vi "GageTransfer.vi"(6 "Length (4096)":dbl=4096.0, 7 "Start (0)":dbl, 8 "Segment (1)":u32=1, 9 "Mode (0)":u32 step=1, 10 "Channel (0)":u16 step=1, 11 "Handle Cluster":T1) -> (0 "Error Code":i32, 1 "Actual Length":dbl, 2 "Data_Raw":i32[](array[numeric]), 3 "Actual Start":dbl)   [LabVIEW 2013]
doc: "This VI transfers the data from one channel of the CompuScope system identified by Handle Cluster, which is obtained by calling CsTool-GetSystem.vi. For accurate interpretation of the transferred data, the user should always use the returned Actual Start and Actual Length, and not the requested values. \n\nThis VI can be used for transferring data from 8, 12, 14, and 16 bit CompuScope hardware. Data are transferred from on-board CompuScope memory to PC RAM using PCI Bus Mastering at rates of up to 200 MB/s. \n\nInternally, CsTool-Transfer.vi converts the raw integer ADC code values into double variable voltage values. For more rapid data access, the user may remove the voltage conversion step. The VI will not return programmatic control to LabVIEW until all of the data have been transferred. \n\nIf the call is successful, a 1 is returned in the Error Code indicator. If the call is unsuccessful, an appropriate error code is returned. A descriptive error string may be obtained by calling CsTool-ErrorHandler.vi.\n\n\nInput Value Descriptions:\n\nChannel\nThis integer value specifies the channel from which data are to be transferred. The default value is 0 for the first channel in the CompuScope system. Channels in a LabVIEW CompuScope system begin at 0. If an invalid channel number is given, an error will be returned. Please see the CompuScope hardware manual for more information on channel enumeration.\n\nMode\nThis integer value determines the current transfer mode. Currently, the only valid value for this input is 0.\n\nSegment(1)\nThis integer value determines which Multiple Record segment is to be transferred, if the CompuScope hardware was operating in Multiple Record Mode. For Single Record Mode acquisitions, the user must always set the Record value to 1, which is the default value. If the Record value is too large, an error code will be returned. \n\nStart\nThis double variable value determines the requested starting point of the data transfer from CompuScope memory to PC RAM. Start is specified relative to the trigger address for the acquisition. A Start value of 0 will cause data transfer to begin at the trigger address. Negative Start values are used for the transfer of pre-trigger data. Positive Start values may be used to begin transfer after the trigger address. The default Start value is 0. \n\nLength\nThis double variable value specifies the amount of data, in samples, to be transferred. The default value is 4096. \n\nData in Volts\nThis array variable, of type double, is the LabVIEW buffer variable into which transferred data are returned. The size of the array will be at least Length samples. Data are returned as voltage values, whose conversion depends upon the resolution of the CompuScope system and on the current input range.\n\nActual Start\nThis double variable value returns the actual start point of the data array. The Actual Start may be lower than the requested Start value. This is because the CompuScope memory architecture may force the drivers to download data from an earlier point than the start position. For example, if Start is input to CsTool-Transfer.vi as 0, the Actual Start may return as -2, indicating that two extra samples were returned before the Start position. \n\nThe user must account for the discrepancy between the Start and the Actual Start. The user may choose to ignore samples transferred from before the Start position. Alternatively, the user may conserve these samples, accounting for the fact that the values begin at Actual Start. \n\nActual Length\nThis double variable value returns the actual amount of data transferred, which may be different from the requested Length. The difference, if any, results from CompuScope memory architecture."
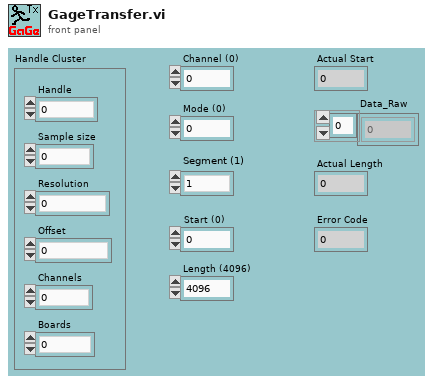
[diagram p1: front panel]
types:
  T1 = cluster{"Handle":u32, "Sample size":u32, "Resolution":i32, "Offset":i32, "Channels":u32, "Boards":u32}
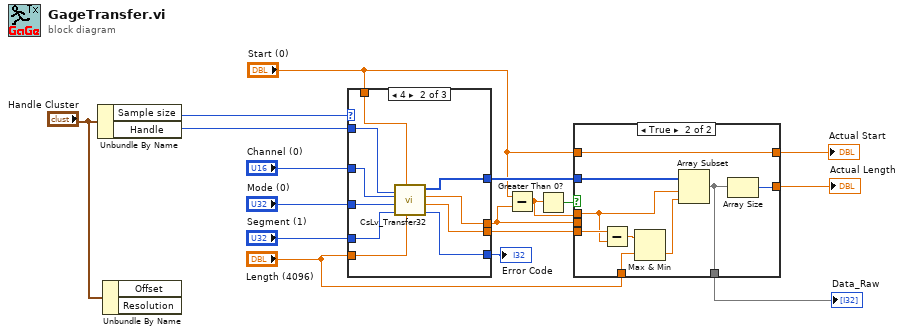
[diagram p0: block diagram]
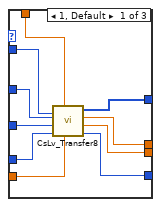
[diagram p3: hidden frame]
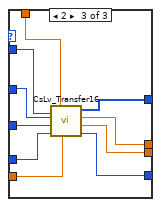
[diagram p4: hidden frame]
diagram:
  n1 = Unbundle By Name("Handle Cluster") -> ("Sample size"=w17:u32, "Handle"=w15:u32)
  n2 = Unbundle By Name("Handle Cluster") -> ()  [unwired: 2 out]
  n3 = case shown="4" w17 {
    tunnel: "Length (4096)" -> [w27 w34 w47]
    tunnel: "Segment (1)" -> [w20 w35 w40]
    tunnel: "Mode (0)" -> [w19 w36 w39]
    tunnel: "Start (0)" -> [w26 w33 w46]
    tunnel: [w25 w29 w45] -> w5
    tunnel: [w24 w30 w44] -> w12
    tunnel: [w23 w32 w43] -> w9
    tunnel: w15 -> [w22 w37 w42]
    tunnel: [w21 w31 w41] -> w7
    tunnel: "Channel (0)" -> [w18 w28 w38]
    frame 1, Default {
      n4 = call <instrlib>:"CsLv_Transfer8.vi"("Handle"=w22, "Length (4096)"=w27, "Start (0)"=w26, "Segment (1)"=w20, "Mode (0)"=w19, "Channel (0)"=w18) -> ("Error Code"=w24:i32, "Actual Length"=w25:dbl, "Actual Start"=w21:dbl, "Buffer out"=w23:u8[])  [unwired: 2 in]
    }
    frame 4 {
      n5 = call <instrlib>:"CsLv_Transfer32.vi"("Handle"=w37, "Length (4096)"=w34, "Start (0)"=w33, "Segment (1)"=w35, "Mode (16)"=w36, "Channel (0)"=w28) -> ("Error Code"=w30:i32, "Actual Length"=w29:dbl, "Actual Start"=w31:dbl, "Buffer out"=w32:i32[])  [unwired: 2 in]
    }
    frame 2 {
      n6 = call <instrlib>:"CsLv_Transfer16.vi"("Start (0)"=w46, "Length (4096)"=w47, "Handle"=w42, "Segment (1)"=w40, "Mode (0)"=w39, "Channel (0)"=w38) -> ("Error Code"=w44:i32, "Actual Length"=w45:dbl, "Actual Start"=w41:dbl, "Buffer"=w43:i16[])  [unwired: 2 in]
    }
  }
  "Error Code" <- w12
  n7 = Subtract(x="Start (0)", y=w7) -> (x-y=w10:dbl)
  n8 = Greater Than 0?(x=w10) -> (x > 0?=w11:bool)
  n9 = case shown="True" w11 {
    tunnel: w10 -> [_ w56]
    tunnel: [w48 w59] -> w2
    tunnel: w5 -> [w50 w57]
    tunnel: [w50 w58] -> w4
    tunnel: "Length (4096)" -> [_ w53]
    tunnel: w9 -> [w48 w52]
    tunnel: [w49 w51] -> w8
    tunnel: "Start (0)" -> [_ w51]
    tunnel: w7 -> [w49 _]
    frame False {
    }
    frame True {
      n10 = Subtract(x=w57, y=w56) -> (x-y=w55:dbl)
      n11 = Max & Min(x=w55, y=w53) -> (min(x,y)=w54:dbl)  [unwired: 1 out]
      n12 = Array Subset(array=w52, index=w56, length=w54) -> (w59:i32[])
      n13 = Array Size(array=w59) -> (size(s)=w58:i32)
    }
  }
  "Data_Raw" <- w2
  "Actual Length" <- w4
  "Actual Start" <- w8
